vi "loadSettings.vi"(8 "error in (no error)":errorcluster, 10 "Path":path, 11 "PixelflySettings in":refnum<class "PixelflySettings.lvclass">) -> (0 "error out":errorcluster, 3 "PixelflySettings out":refnum<class "PixelflySettings.lvclass">)   [LabVIEW 2011, in "Tools.lvlib" / "Settings.lvlib" / "PixelflySettings.lvclass"]
uses:
  PixelflySettings.lvclass
  PixelflySettings.lvclass/PixelflySettings.ctl
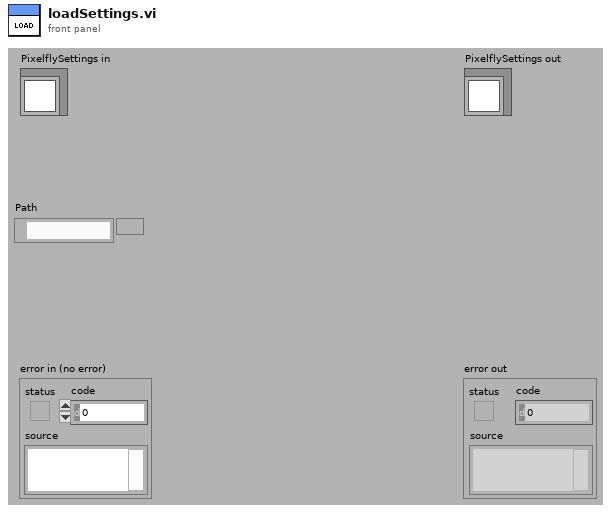
[diagram p1: front panel]
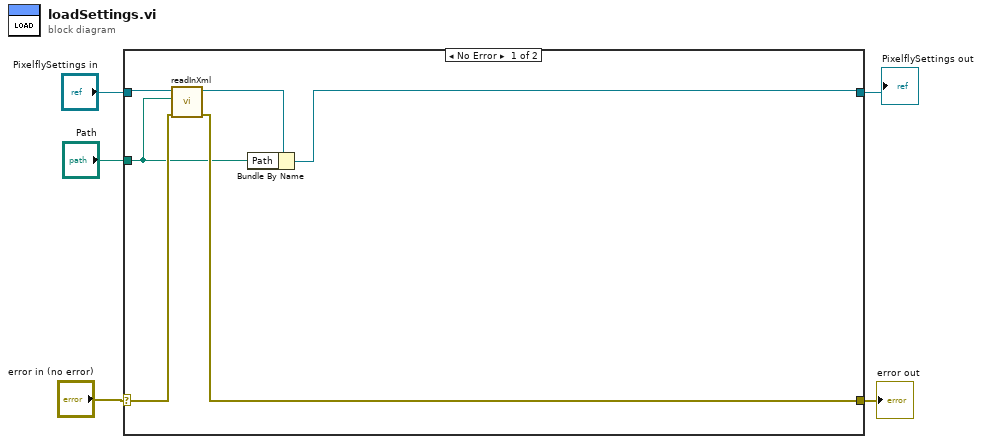
[diagram p0: block diagram]
diagram:
  n1 = case shown="No Error" "error in (no error)" {
    selector: "error in (no error)" -> [w10 w12]
    tunnel: "PixelflySettings in" -> [w11 w13]
    tunnel: [w7 w13] -> w3
    tunnel: [w9 w12] -> w2
    tunnel: "Path" -> [w6 _]
    frame No Error {
      n2 = call "readInXml.vi"("error in (no error)"=w10, "Path"=w6, "PixelflySettings in"=w11) -> ("error out"=w9:errorcluster, "PixelflySettings out"=w8:refnum<class "PixelflySettings.lvclass">)  [unwired: 7 in]
      n3 = Bundle By Name(cluster=w8, "Path"=w6) -> (w7:refnum<class "PixelflySettings.lvclass">)
    }
    frame Error {
    }
  }
  "error out" <- w2
  "PixelflySettings out" <- w3
